vi "CRYGet Legend Name.vi"(10 "MCListbox Refnum":refnum<vi>) -> (3 "Names Out":string[](array[string]))   [LabVIEW 2013]
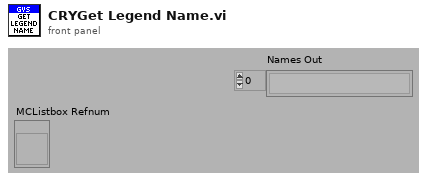
[diagram p1: front panel]
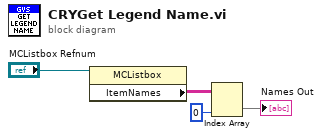
[diagram p0: block diagram]
diagram:
  n1 = property class="MCListbox"(reference="MCListbox Refnum") -> ("ItemNames"=w1:string[][])  [unwired: 1 in, 2 out]
  n2 = Index Array(array=w1, index (col)=0) -> (element=→"Names Out":string[])  [unwired: 1 in]
